vi "Configure Process Value.vi"(0 "VISA resource name":refnum<visa-resource-name>, 1 "Unit Address (1)":u8=1 min=1 max=254, 5 "PV Offset (0)":sgl, 9 "Filter Time Constant (0)":sgl min=0 max=100, 11 "error in (no error)":errorcluster, 14 "Enable Override Filter (False: Disable)":bool) -> (4 "VISA resource name out":refnum<visa-resource-name>, 15 "error out":errorcluster)   [LabVIEW 2010, in "Eurotherm 32xx Series.lvlib"]
doc: "This VI configures process variable parameters."
uses:
  <instrlib>/Eurotherm 32xx Series/Eurotherm 32xx Series.lvlib
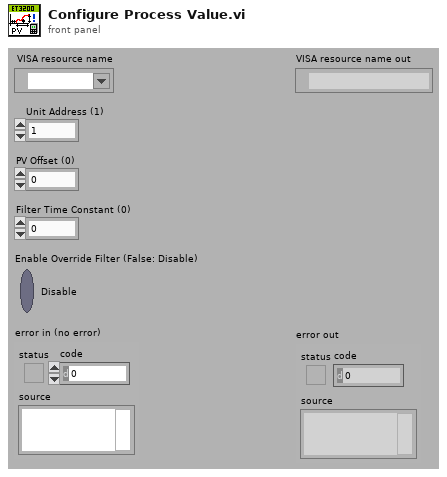
[diagram p1: front panel]
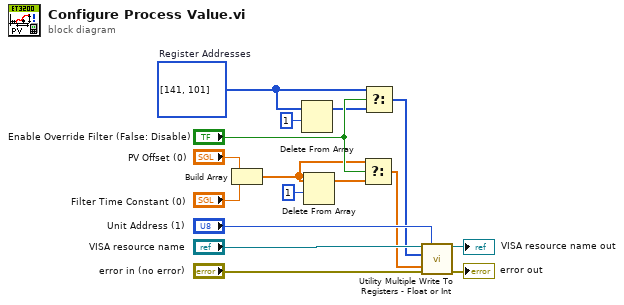
[diagram p0: block diagram]
diagram:
  w4 = i32[] [141, 101]  # Register Addresses
  n1 = Build Array("PV Offset (0)", "Filter Time Constant (0)") -> (w2:sgl[])
  n2 = Delete From Array(array=w4, length=1) -> (array with subset deleted=w3:i32[])  [unwired: 1 in, 1 out]
  n3 = Delete From Array(array=w2, length=1) -> (array with subset deleted=w1:sgl[])  [unwired: 1 in, 1 out]
  n4 = Select(t=w2, s="Enable Override Filter (False: Disable)", f=w1) -> (s? t:f=w6:sgl[])
  n5 = Select(t=w4, s="Enable Override Filter (False: Disable)", f=w3) -> (s? t:f=w7:i32[])
  n6 = call <instrlib>:"Utility Multiple Write To Registers - Float or Int.vi"("VISA resource name"="VISA resource name", "Unit Address (1)"="Unit Address (1)", "Registers Addresses (0)"=w7, "Data (0)"=w6, "error in (no error)"="error in (no error)") -> ("VISA resource name out"=→"VISA resource name out":refnum<visa-resource-name>, "error out"=→"error out":errorcluster)  [unwired: 9 in]
